vi "Util_GetLibUsage.vi"() -> (0 "LibUsage_ProfiledPID":i32 format="%20.0f", 1 "LibUsage_PIDController":i32 format="%20.0f", 2 "LibUsage_Odometry":i32 format="%20.0f", 3 "LibUsage_LinearFIlter":i32 format="%20.0f", 4 "LibUsage_TrapezoidProfile":i32 format="%20.0f", 5 "LibUsage_Kinematics":i32 format="%20.0f")   [LabVIEW 2019, in "Trajectory_Library.lvlib"]
doc: "Returns how many instances of some of the systems in this library are used. The count increments the first time a \"new\" routine is called for a particular pre-allocated clone or inline invocation of a system."
uses:
  Trajectory_Library.lvlib
  Util_LibraryGlobals.vi
panel:
  # "Could add -- SlewRateFilter, MedianFilter, Ramsete, various Feedforward,\n                        Trajectory, Spline."
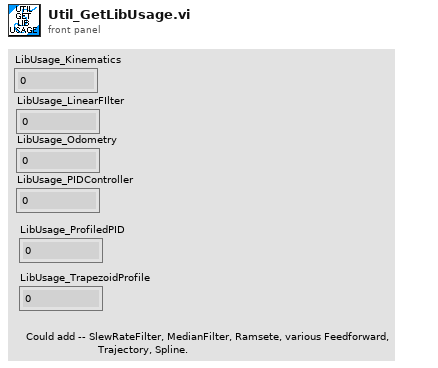
[diagram p1: front panel]
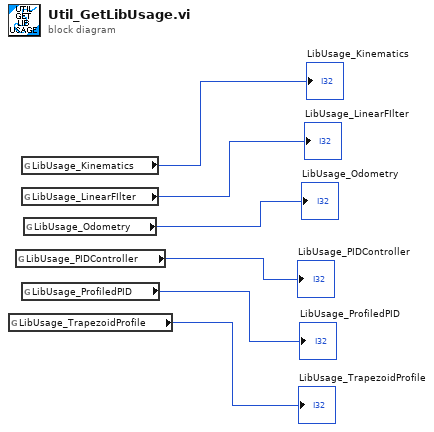
[diagram p0: block diagram]
diagram:
  n1 = global read "Util_LibraryGlobals.vi" "LibUsage_TrapezoidProfile"() -> (→"LibUsage_TrapezoidProfile":i32)
  n2 = global read "Util_LibraryGlobals.vi" "LibUsage_PIDController"() -> (→"LibUsage_PIDController":i32)
  n3 = global read "Util_LibraryGlobals.vi" "LibUsage_Kinematics"() -> (→"LibUsage_Kinematics":i32)
  n4 = global read "Util_LibraryGlobals.vi" "LibUsage_LinearFIlter"() -> (→"LibUsage_LinearFIlter":i32)
  n5 = global read "Util_LibraryGlobals.vi" "LibUsage_ProfiledPID"() -> (→"LibUsage_ProfiledPID":i32)
  n6 = global read "Util_LibraryGlobals.vi" "LibUsage_Odometry"() -> (→"LibUsage_Odometry":i32)
